vi "UDP模拟量发送接收.vi"(10 "第几组":i32) -> (0 "异常_找到?":bool, 1 "接收超时?":bool, 2 "接收的一帧数据":u16[](array[numeric]), 3 "正常_找到?":bool)   [LabVIEW 2010]
uses:
  全局量/全局_配置.vi
panel:
  out "开始时间":dbl format="%#.0f"
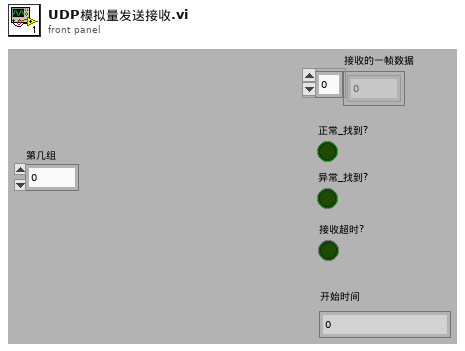
[diagram p1: front panel]
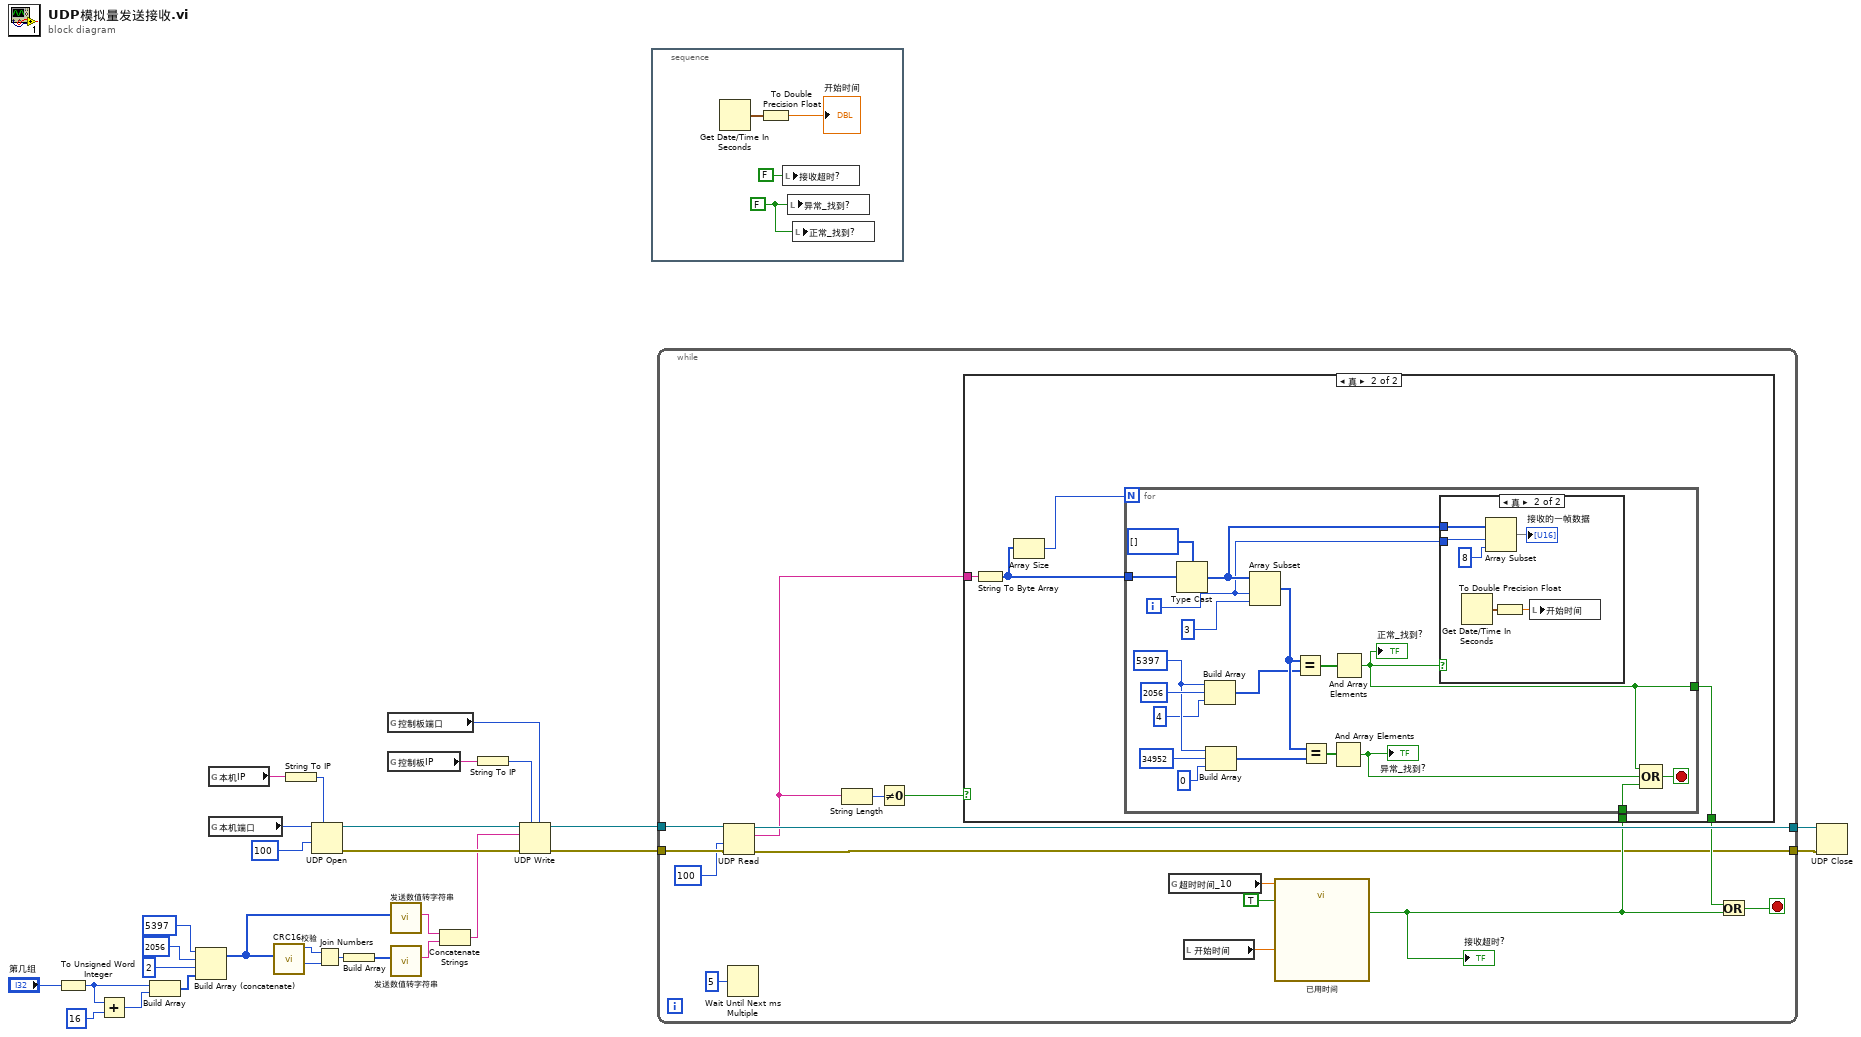
[diagram p0: block diagram]
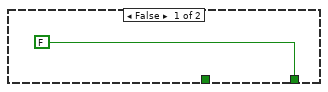
[diagram p2: hidden frame]
diagram:
  n1 = To Unsigned Word Integer(number="第几组") -> (unsigned 16bit integer=w13:u16)
  n2 = Add(x=w13, y=u16 16) -> (x+y=w12:u16)
  n3 = Build Array(w13, w12) -> (w9:u16[])
  n4 = Build Array (concatenate)(u16 5397, u16 2056, u16 2, w9) -> (w23:u16[])
  n5 = global read "全局_配置.vi" "本机IP"() -> (w27:string)
  n6 = global read "全局_配置.vi" "本机端口"() -> (w25:u16)
  n7 = call "CRC16校验.vi"("输入数据_U16"=w23) -> ("低字节"=w18:u8, "高字节"=w17:u8)  [unwired: 9 in]
  n8 = String To IP(1:w27) -> (0:w26:u32)
  n9 = UDP Open(7:w26, 9:100 ("超时毫秒(25000)"), 11:w25) -> (port=w7:refnum<k16>, 0:w6:errorcluster)  [unwired: 2 in, 1 out]
  n10 = Join Numbers(hi=w17, lo=w18) -> ((hi.lo)=w21:u16)
  n11 = Build Array(w21) -> (w22:u16[])
  n12 = global read "全局_配置.vi" "控制板端口"() -> (w2:u16)
  n13 = global read "全局_配置.vi" "控制板IP"() -> (w8:string)
  n14 = call "发送数值转字符串.vi"("输入数据_U16"=w23) -> ("字符串"=w19:string)  [unwired: 10 in]
  n15 = call "发送数值转字符串.vi"("输入数据_U16"=w22) -> ("字符串"=w20:string)  [unwired: 10 in]
  n16 = Concatenate Strings(w19, w20) -> (w1:string)
  n17 = String To IP(1:w8) -> (0:w3:u32)
  n18 = UDP Write(address=w3, port or service name=w2, connection ID=w7, data in=w1, 8:w6) -> (error out=w4:errorcluster, 3:w5:refnum<k16>)  [unwired: 1 in]
  n19 = stacked-sequence {
    frame #0 {
      w31 = FALSE ("找到?")
      n20 = Get Date/Time In Seconds() -> (seconds since 1Jan1904=w33:timestamp)
      n21 = To Double Precision Float(number=w33) -> (double precision float=→"开始时间":dbl)
      n22 = local write "接收超时?"(FALSE ("接收超时?")) -> ()
      n23 = local write "异常_找到?"(w31) -> ()
      n24 = local write "正常_找到?"(w31) -> ()
    }
  }
  n25 = while {
    tunnel: w5 -> [w48]
    tunnel: w4 -> [w47]
    tunnel: [w46] -> w29
    tunnel: [w34] -> w28
    stop <- w38 stop-if-true
    n26 = UDP Read(connection ID=w48, timeout ms (25000)=100, 8:w47) -> (data out=w37:string, error out=w34:errorcluster, 3:w46:refnum<k16>)  [unwired: 1 in, 2 out]
    n27 = Wait Until Next ms Multiple(millisecond multiple=u32 5 ("毫秒倍数")) -> ()  [unwired: 1 out]
    n28 = String Length(string=w37) -> (length=w44:i32)
    n29 = Not Equal To 0?(x=w44) -> (x != 0?=w43:bool)
    n30 = global read "全局_配置.vi" "超时时间_10"() -> (w41:dbl)
    n31 = local read "开始时间"() -> (w40:dbl)
    n32 = call "已用时间"("Time Target (s)"=w41, "Reset"=TRUE, "Set Start Time (s)"=w40) -> ("Time has Elapsed"=w35:bool)  [unwired: 9 in, 7 out]
    "接收超时?" <- w35
    n33 = case shown="真" w43 {
      tunnel: w37 -> [_ w53]
      tunnel: [FALSE ("找到?") w54] -> w39
      tunnel: w35 -> [_ w52]
      frame False {
      }
      frame True {
        n34 = String To Byte Array(string=w53) -> (unsigned byte array=w51:u8[])
        n35 = Array Size(array=w51) -> (size(s)=w50:i32)
        n36 = for {
          N: w50 -> [_]
          tunnel: w51 -> [w73]
          tunnel: [w55] -> w54
          tunnel: w52 -> [w63]
          i -> [w66]
          stop <- w65 stop-if-true
          w61 = u16 5397
          n37 = Type Cast(type=u16[] [], x=w73) -> (*(type *) &x=w67:u16[])
          n38 = Build Array(w61, u16 2056, u16 4) -> (w57:u16[])
          n39 = Build Array(w61, u16 34952, u16 0 ("元素")) -> (w56:u16[])
          n40 = Array Subset(array=w67, index=w66, length=3 ("长度")) -> (w68:u16[])
          n41 = Equal?(x=w68, y=w57) -> (x = y?=w69:bool[])
          n42 = Equal?(x=w68, y=w56) -> (x = y?=w70:bool[])
          n43 = And Array Elements(Boolean array=w70) -> (logical AND=w64:bool)
          "异常_找到?" <- w64
          n44 = And Array Elements(Boolean array=w69) -> (logical AND=w55:bool)
          "正常_找到?" <- w55
          n45 = case shown="真" w55 {
            tunnel: w67 -> [_ w79]
            tunnel: w66 -> [_ w78]
            frame False {
            }
            frame True {
              n46 = Get Date/Time In Seconds() -> (seconds since 1Jan1904=w76:timestamp)
              n47 = Array Subset(array=w79, index=w78, length=8 ("长度")) -> (→"接收的一帧数据":u16[])
              n48 = To Double Precision Float(number=w76) -> (double precision float=w75:dbl)
              n49 = local write "开始时间"(w75) -> ()
            }
          }
          n50 = Compound Arithmetic op=OR(w55, w64, w63) -> (w65:bool)
        }
      }
    }
    n51 = Or(x=w39, y=w35) -> (x .or. y?=w38:bool)
  }
  n52 = UDP Close(connection ID=w29, 8:w28) -> ()  [unwired: 2 out]
